vi "Setup.vi"(11 "TEMPLATE Event in":refnum<class "TEMPLATE Event.lvclass">) -> (3 "TEMPLATE Event out":refnum<class "TEMPLATE Event.lvclass">)   [LabVIEW 2021, in "_Template.lvlib" / "Templates.lvlib" / "TEMPLATE Event.lvlib" / "TEMPLATE Event.lvclass"]
uses:
  TEMPLATE Event.lvclass
  TEMPLATE Event.lvclass/TEMPLATE Event.ctl
  jettl/jettl/Event/Event.lvclass
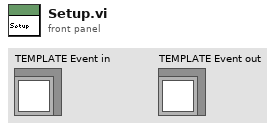
[diagram p1: front panel]
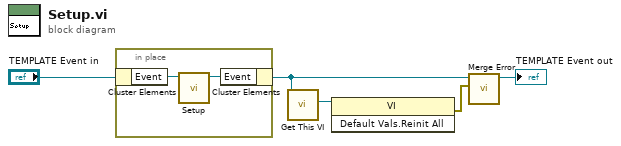
[diagram p0: block diagram]
diagram:
  n1 = in-place {
    n2 = in-place-cluster #1("TEMPLATE Event in") -> ("Event"=w7:refnum<class "Event.lvclass">)
    n3 = call-dynamic "Setup.vi"("Setup in"=w7) -> ("Setup out"=w6:refnum<class "Event.lvclass">)  [unwired: 10 in]
    n4 = in-place-cluster #1("Event"=w6) -> (w2:refnum<class "TEMPLATE Event.lvclass">)
  }
  n5 = call-dynamic "Get This VI.vi"("TEMPLATE Event in"=w2) -> ("This VI"=w4:refnum<vi>)  [unwired: 10 in]
  n6 = invoke class="VI" method="Default Vals.Reinit All"(reference=w4) -> (error out=w3:errorcluster)  [unwired: 2 in, 2 out]
  n7 = call-dynamic "Merge Error.vi"("Error"=w3, "TEMPLATE Event in"=w2) -> ("TEMPLATE Event out"=→"TEMPLATE Event out":refnum<class "TEMPLATE Event.lvclass">)  [unwired: 9 in]
